vi "Robolog.vi"(6 "custom data":string, 9 "Binding Refnum":refnum<notifier>, 10 "Window Mode Notifier":refnum<notifier>) -> (2 "JSON Output":string)   [LabVIEW 2014]
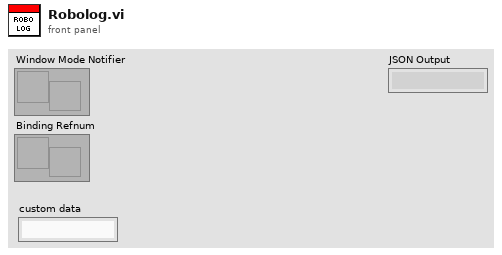
[diagram p1: front panel]
types:
  T1 = cluster{"Error Strings":string, "Disable Counts":cluster{u16, u16}, "Rail Faults":cluster{u16, u16, u16}, "Robot IP":string, "DB Mode":u8, "Event Info":cluster{"Name":string, "Type":u8, "Number":u16, "Replay":u8}, "Camera Addr":string}
  T2 = cluster{"Storage":cluster{"Disk Free":u64, "RAM Block":u32, "RAM free":u32}, "CPU Utilization":cluster{"CPU % ISR":sgl, "CPU % Time Crit":sgl, "CPU % Timed Str":sgl, "CPU % High":sgl, "CPU % Above":sgl, "CPU % Normal":sgl, "CPU % Low":sgl}, "CAN":cluster{"% Bus Utilization":sgl, "Bus Off Cnt":u32, "TX_FIFO Full Cnt":u32, "Receive Error Cnt":u8, "Transmit Error Cnt":u8}, "HID":cluster{"HID Outputs":u32, "Rumble Low":u16, "Rumble High":u16}[]}
  T3 = cluster{"Status bits":cluster{"Test Mode":bool, "Autonomous":bool, "Enabled":bool, "Code Start":bool, "Brownout":bool, "Reserved 2":bool, "Reserved 3":bool, "E-Stop":bool}, "Code Trace":cluster{"Disabled":bool, "TeleOp":bool, "Auto":bool, "Test":bool}, "Controller Type":enum16{"unknown", "cRIO", "roboRio"}, "Code?":enum16{"unknown", "noCode", "code"}, "Battery V":dbl}
  T4 = cluster{"Control Bits":cluster{"TestMode":bool, "Autonomous":bool, "Enabled":bool, "FMS Present":bool, bool, bool, bool, "E-Stop":bool}, "Team Station ":u8, "Countdown":sgl, "Joystick Values":cluster{"Axes":dbl[], "Buttons":bool[], "POVs":i16[]}[]}
  T5 = cluster{"TestMode":bool, "Autonomous":bool, "Enabled":bool, "FMS Present":bool, bool, bool, bool, "E-Stop":bool}
  T6 = cluster{"Test Mode":bool, "Autonomous":bool, "Enabled":bool, "Code Start":bool, "Brownout":bool, "Reserved 2":bool, "Reserved 3":bool, "E-Stop":bool}
  T7 = cluster{"Disabled":bool, "TeleOp":bool, "Auto":bool, "Test":bool}
  T8 = cluster{"Name":string, "Type":u8, "Number":u16, "Replay":u8}
  T9 = cluster{"Disk Free":u64, "RAM Block":u32, "RAM free":u32}
  T10 = cluster{"CPU % ISR":sgl, "CPU % Time Crit":sgl, "CPU % Timed Str":sgl, "CPU % High":sgl, "CPU % Above":sgl, "CPU % Normal":sgl, "CPU % Low":sgl}
  T11 = cluster{"% Bus Utilization":sgl, "Bus Off Cnt":u32, "TX_FIFO Full Cnt":u32, "Receive Error Cnt":u8, "Transmit Error Cnt":u8}
  T12 = cluster{"HID Outputs":u32, "Rumble Low":u16, "Rumble High":u16}[]
  T13 = cluster{"HID Outputs":u32, "Rumble Low":u16, "Rumble High":u16}
  T14 = enum16{"open", "open or create", "create or replace", "create", "open (read only)"}
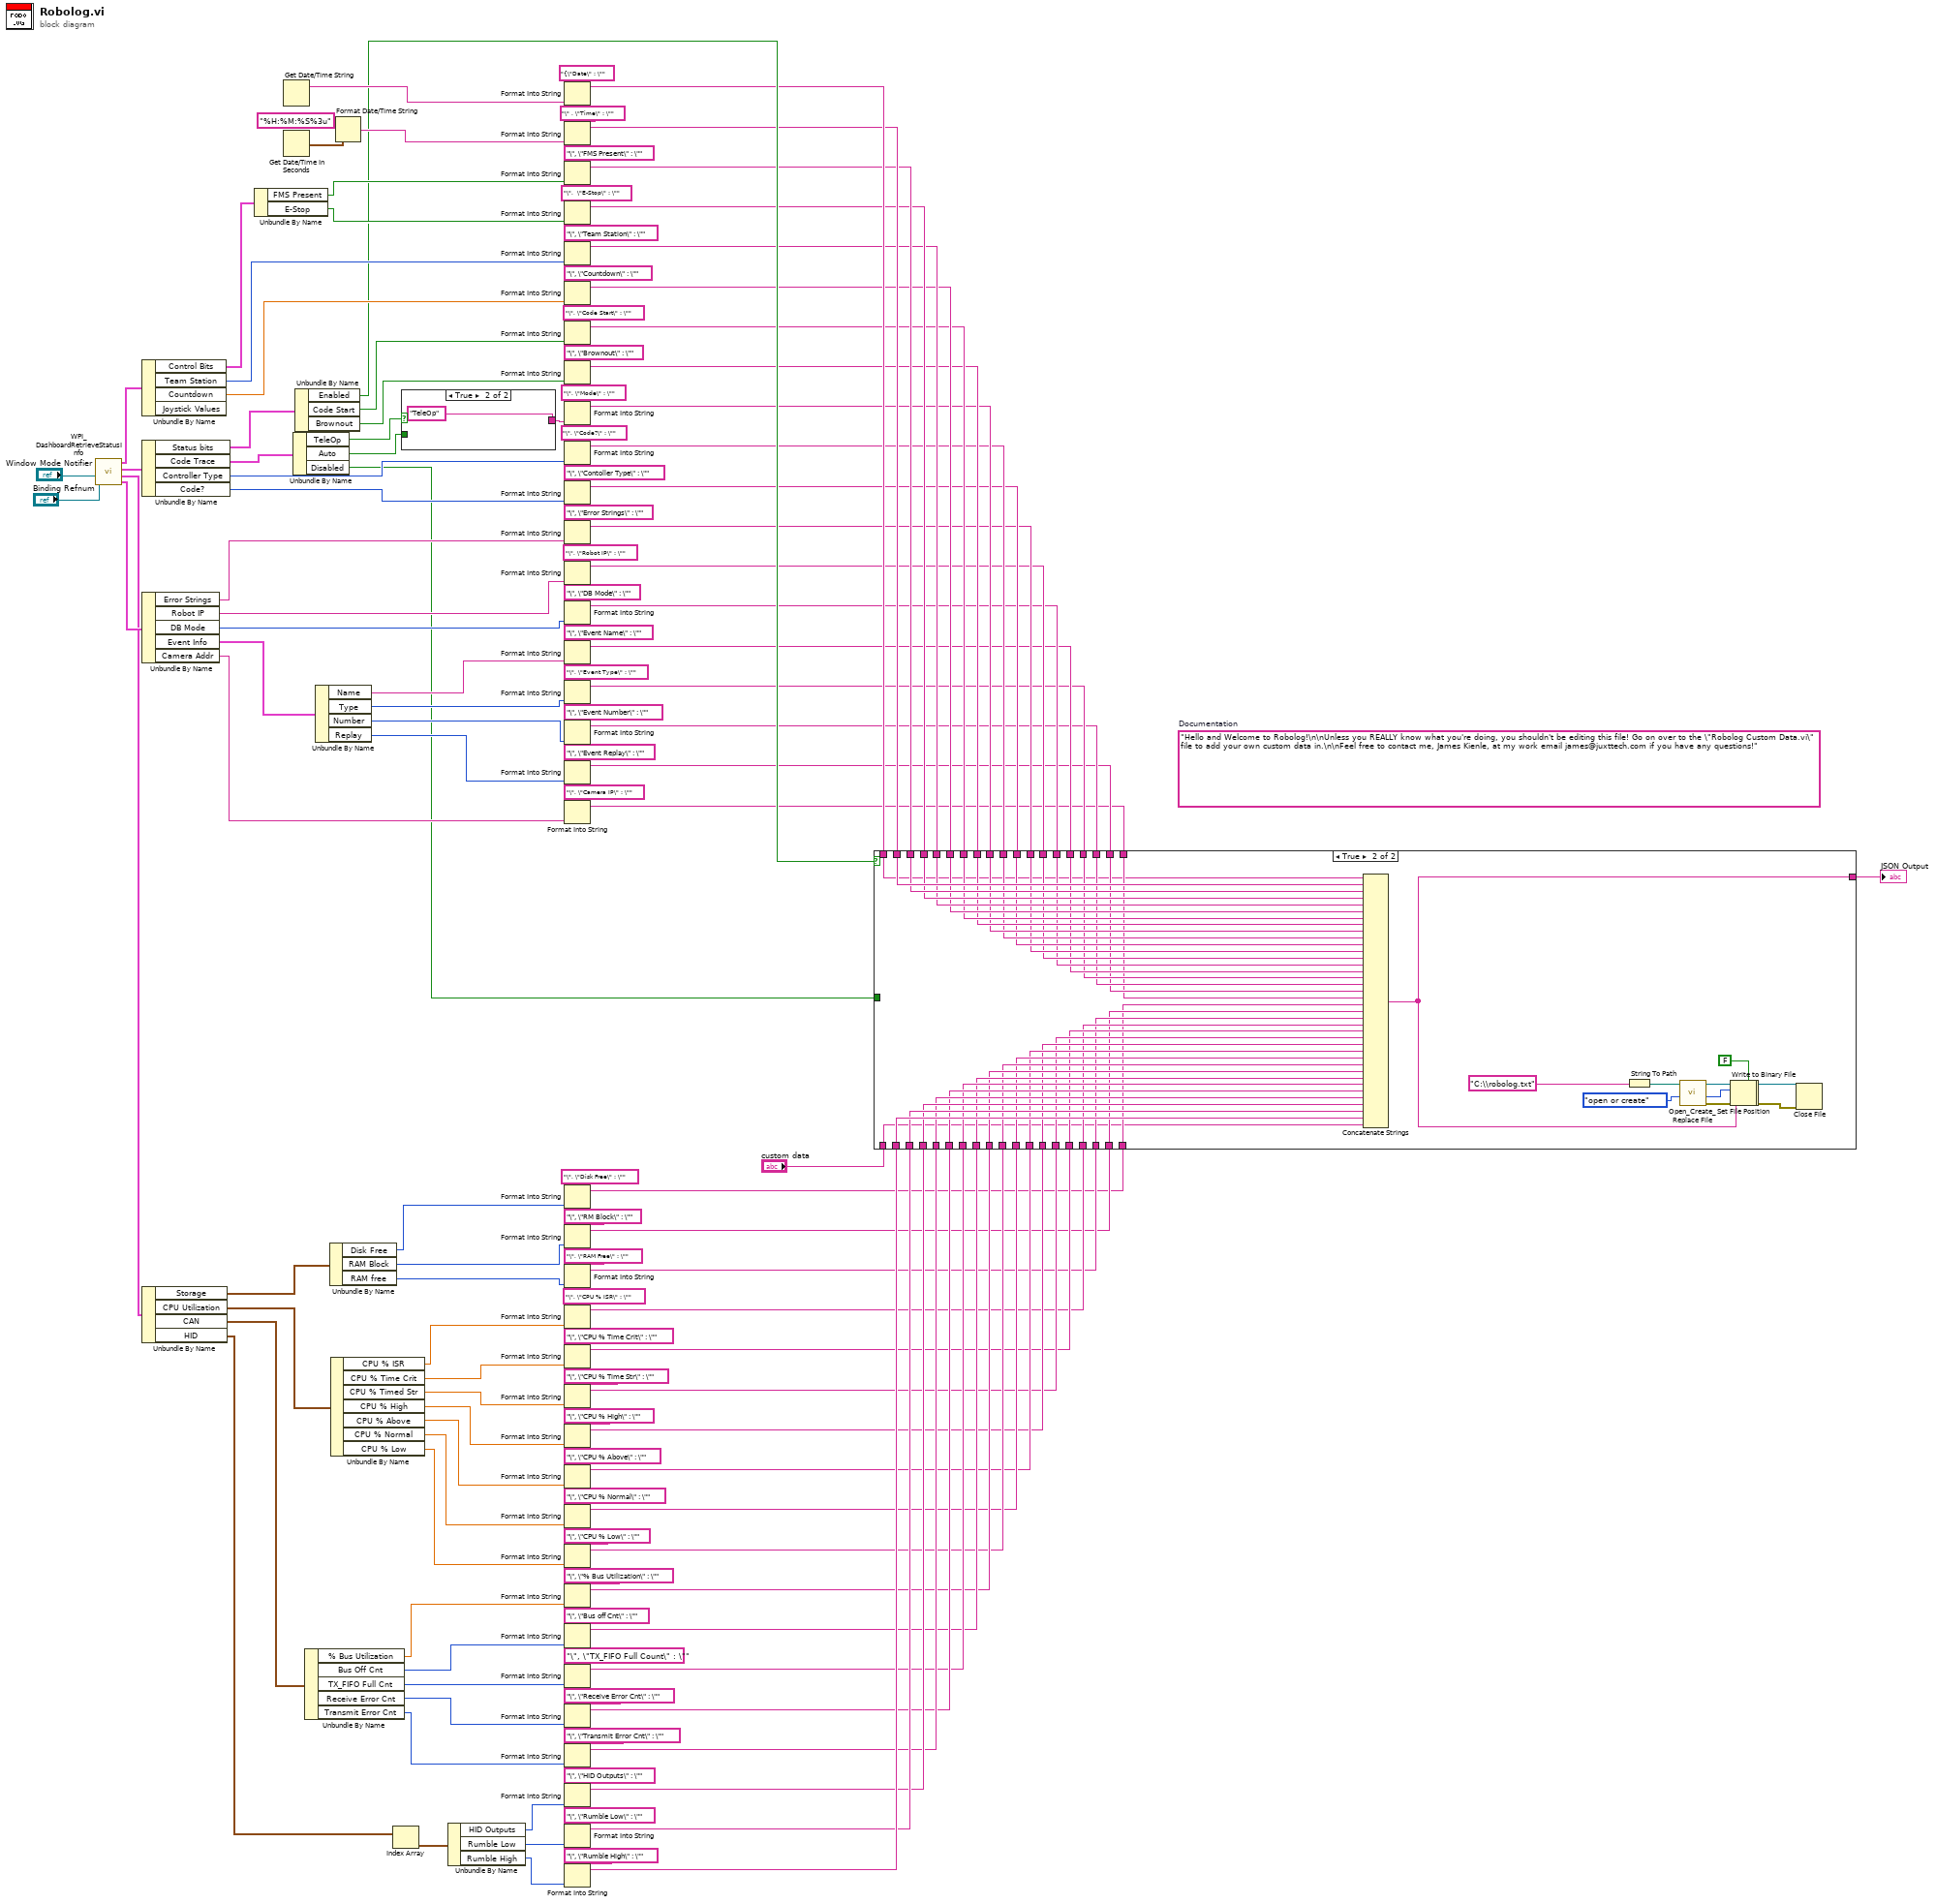
[diagram p0: block diagram]
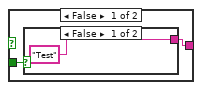
[diagram p2: hidden frame]
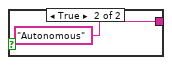
[diagram p3: hidden frame]
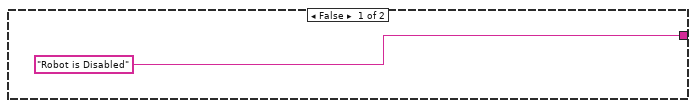
[diagram p4: hidden frame]
diagram:
  (unwired) "Hello and Welcome to Robolog!\n\nUnless you REALLY know what you're doing, you shouldn't be editing this file! Go on over to the \"Robolog Custom Data.vi\" file to add your own custom data in.\n\nFeel free to contact me, James Kienle, at my work email james@juxttech.com if you have any questions!"  # Documentation
  n1 = call <vilib>:"WPI_DashboardRetrieveStatusInfo.vi"("Binding Refnum"="Binding Refnum", "Window Mode Notifier"="Window Mode Notifier") -> ("Power and Errors"=w124:T1, "Robot Metrics"=w63:T2, "Status Info"=w125:T3, "Control Info"=w126:T4)  [unwired: 4 in, 2 out]
  n2 = Unbundle By Name(w126) -> ("Control Bits"=w134:T5, "Team Station"=w130:u8, "Countdown"=w128:sgl)  [unwired: 1 out]
  n3 = Unbundle By Name(w125) -> ("Status bits"=w127:T6, "Code Trace"=w118:T7, "Controller Type"=w102:enum16{"unknown", "cRIO", "roboRio"}, "Code?"=w101:enum16{"unknown", "noCode", "code"})
  n4 = Unbundle By Name(w124) -> ("Error Strings"=w97:string, "Robot IP"=w98:string, "DB Mode"=w95:u8, "Event Info"=w94:T8, "Camera Addr"=w83:string)
  n5 = Unbundle By Name(w63) -> ("Storage"=w62:T9, "CPU Utilization"=w58:T10, "CAN"=w50:T11, "HID"=w29:T12)
  n6 = Unbundle By Name(w134) -> ("FMS Present"=w108:bool, "E-Stop"=w109:bool)
  n7 = Get Date/Time String() -> (date string=w123:string)  [unwired: 3 in, 1 out]
  n8 = Get Date/Time In Seconds() -> (seconds since 1Jan1904=w122:timestamp)
  n9 = Unbundle By Name(w118) -> ("TeleOp"=w104:bool, "Auto"=w103:bool, "Disabled"=w2:bool)
  n10 = Unbundle By Name(w127) -> ("Enabled"=w93:bool, "Code Start"=w107:bool, "Brownout"=w106:bool)
  n11 = Unbundle By Name(w50) -> ("% Bus Utilization"=w49:sgl, "Bus Off Cnt"=w48:u32, "TX_FIFO Full Cnt"=w47:u32, "Receive Error Cnt"=w46:u8, "Transmit Error Cnt"=w45:u8)
  n12 = Unbundle By Name(w94) -> ("Name"=w91:string, "Type"=w89:u8, "Number"=w87:u16, "Replay"=w85:u8)
  n13 = Unbundle By Name(w62) -> ("Disk Free"=w61:u64, "RAM Block"=w60:u32, "RAM free"=w59:u32)
  n14 = Unbundle By Name(w58) -> ("CPU % ISR"=w57:sgl, "CPU % Time Crit"=w56:sgl, "CPU % Timed Str"=w55:sgl, "CPU % High"=w54:sgl, "CPU % Above"=w53:sgl, "CPU % Normal"=w52:sgl, "CPU % Low"=w51:sgl)
  n15 = Format Date/Time String(time format string (%c)="%H:%M:%S%3u", seconds (now)=w122) -> (date/time string=w111:string)  [unwired: 1 in]
  n16 = Index Array(array=w29) -> (element=w28:T13)  [unwired: 1 in]
  n17 = case shown="True" w104 {
    tunnel: [w136 "TeleOp"] -> w105
    tunnel: w103 -> [w135 _]
    frame False {
      n18 = case shown="False" w135 {
        tunnel: ["Test" "Autonomous"] -> w136
        frame False {
        }
        frame True {
        }
      }
    }
    frame True {
    }
  }
  n19 = Unbundle By Name(w28) -> ("HID Outputs"=w26:u32, "Rumble Low"=w24:u16, "Rumble High"=w22:u16)
  n20 = Format Into String(initial string="{\"Date\" : \"", w123) -> (resulting string=w82:string)  [unwired: 2 in, 1 out]
  n21 = Format Into String(initial string="\" , \"Time\" : \"", w111) -> (resulting string=w81:string)  [unwired: 2 in, 1 out]
  n22 = Format Into String(initial string="\", \"FMS Present\" : \"", w108) -> (resulting string=w80:string)  [unwired: 2 in, 1 out]
  n23 = Format Into String(initial string="\",  \"E-Stop\" : \"", w109) -> (resulting string=w79:string)  [unwired: 2 in, 1 out]
  n24 = Format Into String(initial string="\", \"Team Station\" : \"", w130) -> (resulting string=w78:string)  [unwired: 2 in, 1 out]
  n25 = Format Into String(initial string="\", \"Countdown\" : \"", w128) -> (resulting string=w77:string)  [unwired: 2 in, 1 out]
  n26 = Format Into String(initial string="\", \"Code Start\" : \"", w107) -> (resulting string=w76:string)  [unwired: 2 in, 1 out]
  n27 = Format Into String(initial string="\", \"Brownout\" : \"", w106) -> (resulting string=w75:string)  [unwired: 2 in, 1 out]
  n28 = Format Into String(initial string="\", \"Mode\" : \"", w105) -> (resulting string=w74:string)  [unwired: 2 in, 1 out]
  n29 = Format Into String(initial string="\", \"Code?\" : \"", w102) -> (resulting string=w73:string)  [unwired: 2 in, 1 out]
  n30 = Format Into String(initial string="\", \"Contoller Type\" : \"", w101) -> (resulting string=w72:string)  [unwired: 2 in, 1 out]
  n31 = Format Into String(initial string="\", \"Error Strings\" : \"", w97) -> (resulting string=w71:string)  [unwired: 2 in, 1 out]
  n32 = Format Into String(initial string="\", \"Robot IP\" : \"", w98) -> (resulting string=w70:string)  [unwired: 2 in, 1 out]
  n33 = Format Into String(initial string="\", \"DB Mode\" : \"", w95) -> (resulting string=w69:string)  [unwired: 2 in, 1 out]
  n34 = Format Into String(initial string="\", \"Event Name\" : \"", w91) -> (resulting string=w68:string)  [unwired: 2 in, 1 out]
  n35 = Format Into String(initial string="\", \"Event Type\" : \"", w89) -> (resulting string=w67:string)  [unwired: 2 in, 1 out]
  n36 = Format Into String(initial string="\", \"Event Number\" : \"", w87) -> (resulting string=w66:string)  [unwired: 2 in, 1 out]
  n37 = Format Into String(initial string="\", \"Event Replay\" : \"", w85) -> (resulting string=w65:string)  [unwired: 2 in, 1 out]
  n38 = Format Into String(initial string="\", \"Camera IP\" : \"", w83) -> (resulting string=w64:string)  [unwired: 2 in, 1 out]
  n39 = Format Into String(initial string="\", \"Disk Free\" : \"", w61) -> (resulting string=w4:string)  [unwired: 2 in, 1 out]
  n40 = Format Into String(initial string="\", \"RM Block\" : \"", w60) -> (resulting string=w5:string)  [unwired: 2 in, 1 out]
  n41 = Format Into String(initial string="\", \"RAM Free\" : \"", w59) -> (resulting string=w6:string)  [unwired: 2 in, 1 out]
  n42 = Format Into String(initial string="\", \"CPU % ISR\" : \"", w57) -> (resulting string=w7:string)  [unwired: 2 in, 1 out]
  n43 = Format Into String(initial string="\", \"CPU % Time Crit\" : \"", w56) -> (resulting string=w8:string)  [unwired: 2 in, 1 out]
  n44 = Format Into String(initial string="\", \"CPU % Time Str\" : \"", w55) -> (resulting string=w9:string)  [unwired: 2 in, 1 out]
  n45 = Format Into String(initial string="\", \"CPU % High\" : \"", w54) -> (resulting string=w10:string)  [unwired: 2 in, 1 out]
  n46 = Format Into String(initial string="\", \"CPU % Above\" : \"", w53) -> (resulting string=w11:string)  [unwired: 2 in, 1 out]
  n47 = Format Into String(initial string="\", \"CPU % Normal\" : \"", w52) -> (resulting string=w12:string)  [unwired: 2 in, 1 out]
  n48 = Format Into String(initial string="\", \"CPU % Low\" : \"", w51) -> (resulting string=w13:string)  [unwired: 2 in, 1 out]
  n49 = Format Into String(initial string="\", \"% Bus Utilization\" : \"", w49) -> (resulting string=w14:string)  [unwired: 2 in, 1 out]
  n50 = Format Into String(initial string="\", \"Bus off Cnt\" : \"", w48) -> (resulting string=w15:string)  [unwired: 2 in, 1 out]
  n51 = Format Into String(initial string="\", \"TX_FIFO Full Count\" : \"", w47) -> (resulting string=w16:string)  [unwired: 2 in, 1 out]
  n52 = Format Into String(initial string="\", \"Receive Error Cnt\" : \"", w46) -> (resulting string=w17:string)  [unwired: 2 in, 1 out]
  n53 = Format Into String(initial string="\", \"Transmit Error Cnt\" : \"", w45) -> (resulting string=w18:string)  [unwired: 2 in, 1 out]
  n54 = Format Into String(initial string="\", \"HID Outputs\" : \"", w26) -> (resulting string=w19:string)  [unwired: 2 in, 1 out]
  n55 = Format Into String(initial string="\", \"Rumble Low\" : \"", w24) -> (resulting string=w20:string)  [unwired: 2 in, 1 out]
  n56 = Format Into String(initial string="\", \"Rumble High\" : \"", w22) -> (resulting string=w21:string)  [unwired: 2 in, 1 out]
  n57 = case shown="True" w93 {
    tunnel: w82 -> [_ w172]
    tunnel: w81 -> [_ w190]
    tunnel: w80 -> [_ w189]
    tunnel: w79 -> [_ w188]
    tunnel: w78 -> [_ w187]
    tunnel: w77 -> [_ w186]
    tunnel: w76 -> [_ w185]
    tunnel: w75 -> [_ w184]
    tunnel: w74 -> [_ w183]
    tunnel: w73 -> [_ w182]
    tunnel: w72 -> [_ w181]
    tunnel: w71 -> [_ w180]
    tunnel: w70 -> [_ w179]
    tunnel: w69 -> [_ w178]
    tunnel: w68 -> [_ w177]
    tunnel: w67 -> [_ w176]
    tunnel: w66 -> [_ w175]
    tunnel: w65 -> [_ w174]
    tunnel: w64 -> [_ w173]
    tunnel: w21 -> [_ w171]
    tunnel: w20 -> [_ w170]
    tunnel: w19 -> [_ w169]
    tunnel: w18 -> [_ w168]
    tunnel: w17 -> [_ w167]
    tunnel: w16 -> [_ w166]
    tunnel: w15 -> [_ w165]
    tunnel: w14 -> [_ w164]
    tunnel: w13 -> [_ w163]
    tunnel: w12 -> [_ w162]
    tunnel: w11 -> [_ w161]
    tunnel: w10 -> [_ w160]
    tunnel: w9 -> [_ w159]
    tunnel: w8 -> [_ w158]
    tunnel: w7 -> [_ w157]
    tunnel: w6 -> [_ w156]
    tunnel: w5 -> [_ w155]
    tunnel: w4 -> [_ w154]
    tunnel: "custom data" -> [_ w153]
    tunnel: ["Robot is Disabled" w152] -> w3
    tunnel: w2 -> [_ _]
    frame False {
    }
    frame True {
      n58 = Concatenate Strings(w172, w190, w189, w188, w187, w186, w185, w184, w183, w182, w181, w180, w179, w178, w177, w176, w175, w174, w173, w154, w155, w156, w157, w158, w159, w160, w161, w162, w163, w164, w165, w166, w167, w168, w169, w170, w171, w153) -> (w152:string)
      n59 = String To Path(string="C:\\robolog.txt") -> (path=w142:path)
      n60 = call <vilib>:"Open_Create_Replace File.vi"("function (open:0)"=T14."open or create", "file path"=w142) -> ("error out"=w150:errorcluster, "file size (bytes)"=w148:i32, "refnum"=w149:refnum<file>)  [unwired: 6 in, 1 out]
      n61 = Set File Position(offset (in bytes) (0)=w148, refnum=w149, error in=w150) -> (refnum out=w145:refnum<file>, error out=w144:errorcluster)  [unwired: 1 in]
      n62 = Write to Binary File(file (use dialog)=w145, data=w152, error in=w144, 5:FALSE ("prepend array or string size? (T)")) -> (refnum out=w146:refnum<file>, error out=w147:errorcluster)  [unwired: 2 in, 1 out]
      n63 = Close File(refnum=w146, error in=w147) -> ()  [unwired: 2 out]
    }
  }
  "JSON Output" <- w3
